vi "Get Spectral Map (DBL).vi"(6 "window info":T1={"window type"=10, "window length"=2048} {"window type" items=["None"=0, "Hanning"=1, "Hamming"=2, "Blackman-Harris"=3, "Exact Blackman"=4, "Blackman"=5, "Flat Top"=6, "4 Term B-Harris"=7, "7 Term B-Harris"=8, "Low Sidelobe"=9, "Gaussian"=62]; "window length" min=0}, 7 "dB On (T)":bool=TRUE, 8 "error in (no error)":errorcluster, 9 "type":T4(ring)=enum."RPM-Order", 10 "speed profile":T5 {"speed [RPM]" format="%.2f"; "time [s]" format="%.2f"}, 11 "scaled signal [EU]":waveform(dbl)={"t0"=timestamp(0 s since 1904-01-01), "dt"=0.0, "Y"=[]}) -> (0 "error out":errorcluster, 1 "unit labels":T2, 2 "scales":T3 {"Z scale"."multiplier" format="%.2f"; "Z scale"."offset" format="%.2f"; "Y scale"."multiplier" format="%.2f"; "Y scale"."offset" format="%.2f"; "X scale"."multiplier" format="%.2f"; "X scale"."offset" format="%.2f"}, 3 "spectral map":dbl[][](array[numeric]) format="%.2f", 4 "actual window":T1={"window type"=10, "window length"=2048} {"window type" items=["None"=0, "Hanning"=1, "Hamming"=2, "Blackman-Harris"=3, "Exact Blackman"=4, "Blackman"=5, "Flat Top"=6, "4 Term B-Harris"=7, "7 Term B-Harris"=8, "Low Sidelobe"=9, "Gaussian"=62]; "window length" min=0})   [LabVIEW 2017]
doc: "Returns the spectral map of <B>scaled signal [EU]</B>. You can use this polymorphic VI to return <B>spectral map</B> as a 2D array of double-precision, floating-point numbers or a 2D array of 8-bit unsigned integers. You must manually select the polymorphic instance to use. Use the DBL instance to obtain more accurate data. Use the U8 instance to reduce memory usage when the VI displays data."
uses:
  <vilib>/addons/Sound and Vibration/Order Analysis/Tach Process/SubVIs/speed profile.ctl
  <vilib>/addons/Sound and Vibration/Order Analysis/Ref Gabor Order Tracking/window information.ctl
  <vilib>/addons/Sound and Vibration/Order Analysis/Ref Gabor Order Tracking/Get Order-RPM Spectral Map (DBL).vi
  <vilib>/addons/Sound and Vibration/Order Analysis/Ref Gabor Order Tracking/Get Freq-RPM Spectral Map (DBL).vi
  <vilib>/addons/Sound and Vibration/Order Analysis/Ref Gabor Order Tracking/Get Freq-Time Spectral Map (DBL).vi
  <vilib>/addons/_NISVFA/_Shared subVIs/Common/svc_Engineering Units to Unit Label.vi
  <vilib>/addons/_NISVFA/_Shared subVIs/Common/svc_Unit Label to Engineering Units.vi
  <vilib>/addons/Sound and Vibration/Order Analysis/Gabor Order Tracking/SoundVib_Gabor.lvlib
  <vilib>/addons/Sound and Vibration/Order Analysis/Tach Process/SoundVib_TachProcess.lvlib
panel:
  # "Get Spectral Map (DBL)"
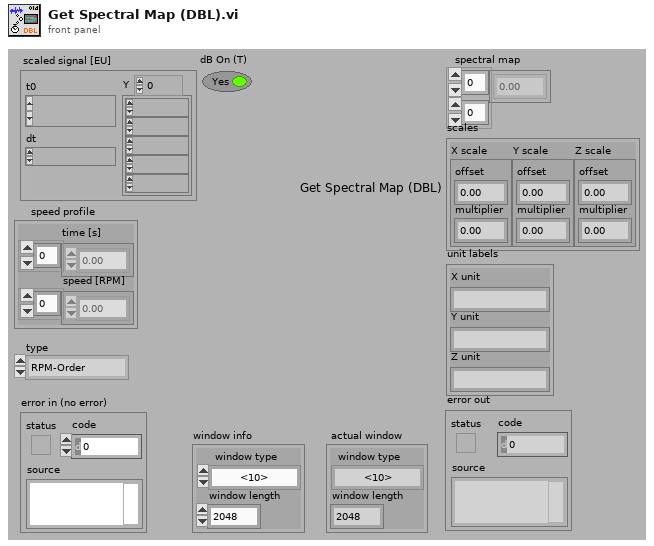
[diagram p1: front panel]
types:
  T1 = typedef "SoundVib_Gabor.lvlib/window information.ctl" = cluster{"window type":u32, "window length":i32}
  T2 = cluster{"X unit":string, "Y unit":string, "Z unit":string}
  T3 = cluster{"X scale":cluster{"offset":dbl, "multiplier":dbl}, "Y scale":cluster{"offset":dbl, "multiplier":dbl}, "Z scale":cluster{"offset":dbl, "multiplier":dbl}}
  T4 = enum16{"Frequency-Time", "Frequency-RPM", "Order-RPM", "RPM-Order"}
  T5 = typedef "SoundVib_TachProcess.lvlib/speed profile.ctl" = cluster{"time [s]":dbl[], "speed [RPM]":dbl[]}
  T6 = typedef "svc_Channel Info.ctl" = cluster{"sensor sensitivity":dbl, "engineering units":T7, "dB reference":dbl, "custom label":string, "weighting filter":T8, "pregain":dbl}
  T7 = typedef "svc_Engineering Units Text Ring.ctl" = u16
  T8 = typedef "svc_Weighting Filter Text Ring.ctl" = u16
  T9 = typedef "SoundVib_Gabor.lvlib/GT RefNum.ctl" = refnum<k1>
  T10 = cluster{"column unit":string, "row unit":string, "unit label":string}
  T11 = cluster{"order scale":cluster{"offset":dbl, "multiplier":dbl}, "rpm scale":cluster{"offset":dbl, "multiplier":dbl}, "quantization info":cluster{"offset":dbl, "multiplier":dbl}}
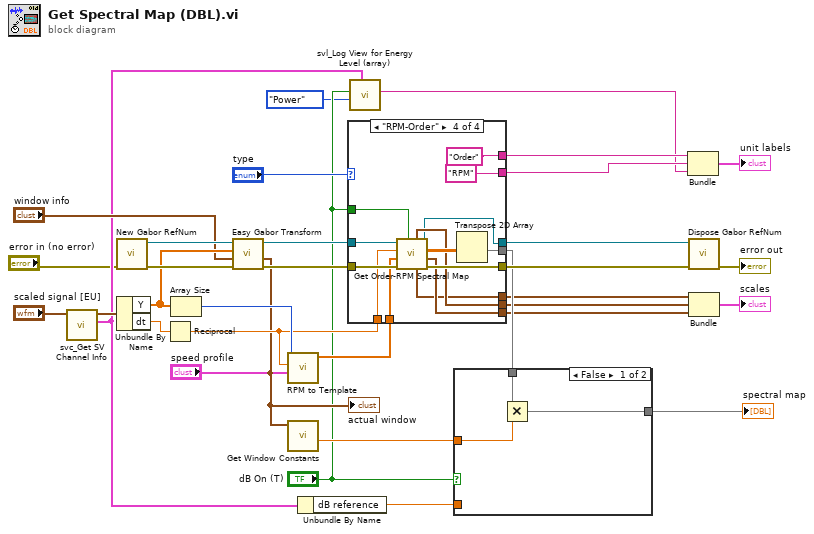
[diagram p0: block diagram]
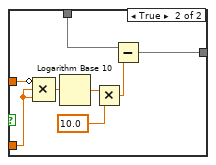
[diagram p2: hidden frame]
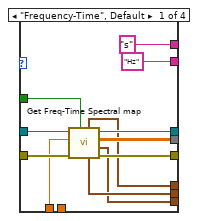
[diagram p3: hidden frame]
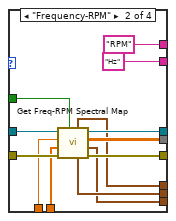
[diagram p4: hidden frame]
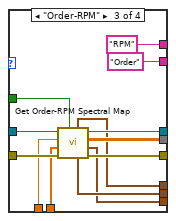
[diagram p5: hidden frame]
diagram:
  n1 = call <vilib>:"svc_Get SV Channel Info.vi"("scaled signal [EU]"="scaled signal [EU]") -> ("channel info"=w4:T6, "dup scaled signal [EU]"=w14:waveform(dbl))  [unwired: 5 in, 4 out]
  n2 = call <vilib>:"New Gabor RefNum.vi"("error in (no error)"="error in (no error)") -> ("error out"=w33:errorcluster, "RefNum"=w34:T9)  [unwired: 8 in]
  n3 = Unbundle By Name(w14) -> ("Y"=w20:dbl[], "dt"=w18:dbl)
  n4 = Reciprocal(x=w18) -> (1/x=w19:dbl)
  n5 = Array Size(array=w20) -> (size(s)=w27:i32)
  n6 = call <vilib>:"Easy Gabor Transform.vi"("error in (no error)"=w33, "window info"="window info", "x[n]"=w20, "RefNum in"=w34) -> ("error out"=w30:errorcluster, "actual window"=w13:T1, "RefNum out"=w31:T9)  [unwired: 3 in, 2 out]
  "actual window" <- w13
  n7 = call <vilib>:"RPM to Template.vi"("window info"=w13, "speed profile"="speed profile", "sampling frequency [Hz]"=w19, "signal length"=w27) -> ("Gabor template"=w25:dbl[])  [unwired: 6 in, 1 out]
  n8 = call <vilib>:"Get Window Constants.vi"("window info"=w13) -> ("multiply factor"=w12:dbl)  [unwired: 9 in, 1 out]
  n9 = Unbundle By Name(w4) -> ("dB reference"=w3:dbl)
  n10 = case shown="\"RPM-Order\"" "type" {
    tunnel: [w46 w54 w71 w73] -> w32
    tunnel: w31 -> [w45 w58 w65 w82]
    tunnel: w30 -> [w44 w57 w68 w85]
    tunnel: [w43 w56 w69 w86] -> w29
    tunnel: "dB On (T)" -> [w42 w52 w64 w81]
    tunnel: [w38 w53 w63 w76] -> w8
    tunnel: [w41 w55 w70 w78] -> w22
    tunnel: [w40 w59 w72 w77] -> w7
    tunnel: w19 -> [w39 w50 w66 w83]
    tunnel: w25 -> [_ w51 w67 w84]
    tunnel: ["s" ("row unit") "RPM" ("row unit") "RPM" ("row unit") "Order" ("column unit")] -> w11
    tunnel: ["Hz" ("column unit") "Hz" ("column unit") "Order" ("column unit") "RPM" ("row unit")] -> w10
    tunnel: [w35 w47 w60 w80] -> w16
    frame "Frequency-Time", Default {
      n11 = call-poly <vilib>:"Get Freq-Time Spectral map.vi"("dB On (T)"=w42, "error in (no error)"=w44, "sampling frequency [Hz]"=w39, "RefNum in"=w45) -> ("error out"=w43:errorcluster, "quantization info"=w35:cluster{"offset":dbl, "multiplier":dbl}, "spectral map"=w41:dbl[][], "RefNum out"=w46:T9, "frequency scale"=w40:cluster{"offset":dbl, "multiplier":dbl}, "time scale"=w38:cluster{"offset":dbl, "multiplier":dbl})  [unwired: 2 in]
    }
    frame "Frequency-RPM" {
      n12 = call-poly <vilib>:"Get Freq-RPM Spectral Map.vi"("dB On (T)"=w52, "error in (no error)"=w57, "Gabor template"=w51, "sampling frequency [Hz]"=w50, "RefNum in"=w58) -> ("error out"=w56:errorcluster, "quantization info"=w47:cluster{"offset":dbl, "multiplier":dbl}, "spectral map"=w55:dbl[][], "RefNum out"=w54:T9, "frequency scale"=w59:cluster{"offset":dbl, "multiplier":dbl}, "rpm scale"=w53:cluster{"offset":dbl, "multiplier":dbl})  [unwired: 1 in]
    }
    frame "Order-RPM" {
      n13 = call-poly <vilib>:"Get Order-RPM Spectral Map.vi"("dB On (T)"=w64, "error in (no error)"=w68, "Gabor template"=w67, "sampling frequency [Hz]"=w66, "RefNum in"=w65) -> ("error out"=w69:errorcluster, "quantization info"=w60:cluster{"offset":dbl, "multiplier":dbl}, "spectral map"=w70:dbl[][], "RefNum out"=w71:T9, "order scale"=w72:cluster{"offset":dbl, "multiplier":dbl}, "rpm scale"=w63:cluster{"offset":dbl, "multiplier":dbl})  [unwired: 1 in]
    }
    frame "RPM-Order" {
      n14 = call-poly <vilib>:"Get Order-RPM Spectral Map.vi"("dB On (T)"=w81, "error in (no error)"=w85, "Gabor template"=w84, "sampling frequency [Hz]"=w83, "RefNum in"=w82) -> ("error out"=w86:errorcluster, "quantization info"=w80:cluster{"offset":dbl, "multiplier":dbl}, "spectral map"=w79:dbl[][], "RefNum out"=w73:T9, "order scale"=w76:cluster{"offset":dbl, "multiplier":dbl}, "rpm scale"=w77:cluster{"offset":dbl, "multiplier":dbl})  [unwired: 1 in]
      n15 = Transpose 2D Array(2D array=w79) -> (transposed array=w78:dbl[][])
    }
  }
  n16 = call <vilib>:"svl_Log View for Energy Level (array).vi"("channel info"=w4, "view mode"=enum16{"Power", "Amplitude"}."Power", "dB On (T)"="dB On (T)") -> ("unit label"=w5:string)  [unwired: 6 in, 2 out]
  n17 = case shown="False" "dB On (T)" {
    tunnel: w22 -> [w88 w93]
    tunnel: [w89 w94] -> w9
    tunnel: w12 -> [w87 w92]
    tunnel: w3 -> [_ w90]
    frame False {
      n18 = Multiply(x=w88, y=w87) -> (x*y=w89:dbl[][])
    }
    frame True {
      n19 = Compound Arithmetic op=MULTIPLY(invert w92, w90, w90) -> (w91:dbl)
      n20 = Logarithm Base 10(1:w91) -> (0:w96:dbl)
      n21 = Multiply(x=w96, y=10.0) -> (x*y=w95:dbl)
      n22 = Subtract(x=w93, y=w95) -> (x-y=w94:dbl[][])
    }
  }
  "spectral map" <- w9
  n23 = Bundle("column unit"=w11, "row unit"=w10, "unit label"=w5) -> (→"unit labels":T10)  [unwired: 1 in]
  n24 = call <vilib>:"Dispose Gabor RefNum.vi"("error in (no error)"=w29, "RefNum in"=w32) -> ("error out"=→"error out":errorcluster)  [unwired: 6 in]
  n25 = Bundle("order scale"=w8, "rpm scale"=w7, "quantization info"=w16) -> (→"scales":T11)  [unwired: 1 in]
